vi "IRGetLastLearnedCode.vi"(8 "error in (no error)":errorcluster, 11 "Device In":u64) -> (0 "error out":errorcluster, 1 "codeInfo out":T1={"bitCount"=0, "encoding"=1, "length"=1, "gap"=0, "trail"=0, "header[0]"=0, "header[1]"=0, "one[0]"=0, "one[1]"=0, "zero[0]"=0, "zero[1]"=0, "repeat[0]"=0, "repeat[1]"=0, "repeat[2]"=0, "repeat[3]"=0, "repeat[4]"=0, "repeat[5]"=0, "repeat[6]"=0, "repeat[7]"=0, "repeat[8]"=0, "repeat[9]"=0, "repeat[10]"=0, "repeat[11]"=0, "repeat[12]"=0, "repeat[13]"=0, "repeat[14]"=0, "repeat[15]"=0, "repeat[16]"=0, "repeat[17]"=0, "repeat[18]"=0, "repeat[19]"=0, "repeat[20]"=0, "repeat[21]"=0, "repeat[22]"=0, "repeat[23]"=0, "repeat[24]"=0, "repeat[25]"=0, "minRepeat"=0, "dutyCycle"=0.0, "carrierFrequency"=0, "toggleMask[0]"=0, "toggleMask[1]"=0, "toggleMask[2]"=0, "toggleMask[3]"=0, "toggleMask[4]"=0, "toggleMask[5]"=0, "toggleMask[6]"=0, "toggleMask[7]"=0, "toggleMask[8]"=0, "toggleMask[9]"=0, "toggleMask[10]"=0, "toggleMask[11]"=0, "toggleMask[12]"=0, "toggleMask[13]"=0, "toggleMask[14]"=0, "toggleMask[15]"=0, "toggleMask[16]"=0, "toggleMask[17]"=0, "toggleMask[18]"=0, "toggleMask[19]"=0, "toggleMask[20]"=0, "toggleMask[21]"=0, "toggleMask[22]"=0, "toggleMask[23]"=0, "toggleMask[24]"=0, "toggleMask[25]"=0, "toggleMask[26]"=0, "toggleMask[27]"=0, "toggleMask[28]"=0, "toggleMask[29]"=0, "toggleMask[30]"=0, "toggleMask[31]"=0, "toggleMask[32]"=0} caption="Code Info" {"encoding" items=["IR_ENCODING_UNKNOWN"=1, "IR_ENCODING_SPACE"=2, "IR_ENCODING_PULSE"=3, "IR_ENCODING_BIPHASE"=4, "IR_ENCODING_RC5"=5, "IR_ENCODING_RC6"=6]; "length" items=["IR_LENGTH_UNKNOWN"=1, "IR_LENGTH_CONSTANT"=2, "IR_LENGTH_VARIABLE"=3]}, 2 "Learned Code":string, 3 "Device Out":u64)   [LabVIEW 2012, in "Phidget IR.lvlib"]
doc: "${GetLastLearnedCode:Header}"
uses:
  <instrlib>/Phidgets/Phidget IR/Phidget IR.lvlib
  <instrlib>/Phidgets/Phidget IR/Public/CodeInfo.ctl
  <instrlib>/Phidgets/Phidget Common/Phidget Common.lvlib
  phidget22.dll
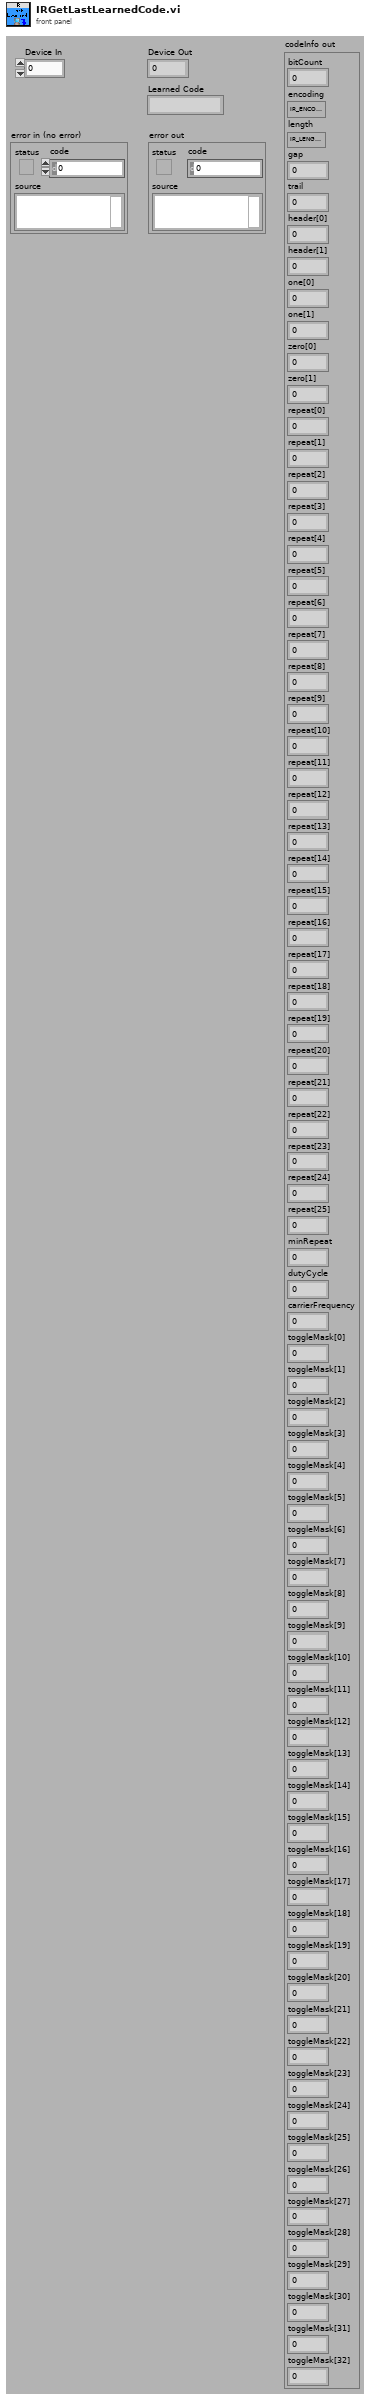
[diagram p1: front panel]
types:
  T1 = typedef "Phidget IR.lvlib/CodeInfo.ctl" = cluster{"bitCount":u32, "encoding":u32, "length":u32, "gap":u32, "trail":u32, "header[0]":u32, "header[1]":u32, "one[0]":u32, "one[1]":u32, "zero[0]":u32, "zero[1]":u32, "repeat[0]":u32, "repeat[1]":u32, "repeat[2]":u32, "repeat[3]":u32, "repeat[4]":u32, "repeat[5]":u32, "repeat[6]":u32, "repeat[7]":u32, "repeat[8]":u32, "repeat[9]":u32, "repeat[10]":u32, "repeat[11]":u32, "repeat[12]":u32, "repeat[13]":u32, "repeat[14]":u32, "repeat[15]":u32, "repeat[16]":u32, "repeat[17]":u32, "repeat[18]":u32, "repeat[19]":u32, "repeat[20]":u32, "repeat[21]":u32, "repeat[22]":u32, "repeat[23]":u32, "repeat[24]":u32, "repeat[25]":u32, "minRepeat":u32, "dutyCycle":dbl, "carrierFrequency":u32, "toggleMask[0]":i8, "toggleMask[1]":i8, "toggleMask[2]":i8, "toggleMask[3]":i8, "toggleMask[4]":i8, "toggleMask[5]":i8, "toggleMask[6]":i8, "toggleMask[7]":i8, "toggleMask[8]":i8, "toggleMask[9]":i8, "toggleMask[10]":i8, "toggleMask[11]":i8, "toggleMask[12]":i8, "toggleMask[13]":i8, "toggleMask[14]":i8, "toggleMask[15]":i8, "toggleMask[16]":i8, "toggleMask[17]":i8, "toggleMask[18]":i8, "toggleMask[19]":i8, "toggleMask[20]":i8, "toggleMask[21]":i8, "toggleMask[22]":i8, "toggleMask[23]":i8, "toggleMask[24]":i8, "toggleMask[25]":i8, "toggleMask[26]":i8, "toggleMask[27]":i8, "toggleMask[28]":i8, "toggleMask[29]":i8, "toggleMask[30]":i8, "toggleMask[31]":i8, "toggleMask[32]":i8}
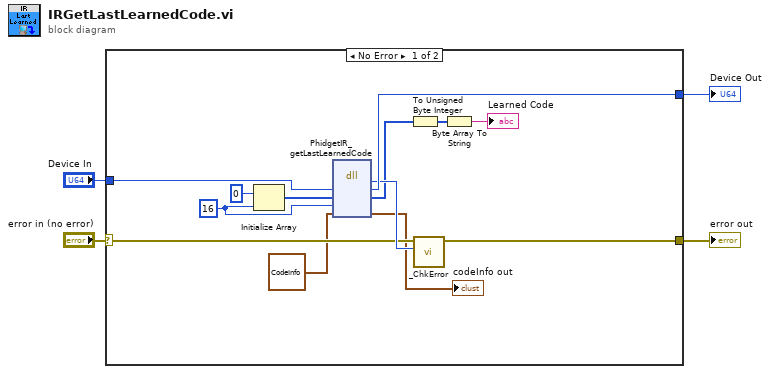
[diagram p0: block diagram]
diagram:
  n1 = case shown="No Error" "error in (no error)" {
    selector: "error in (no error)" -> [w14 w19]
    tunnel: [w13 w19] -> w3
    tunnel: "Device In" -> [w17 w18]
    tunnel: [w16 w18] -> w1
    frame No Error {
      w7 = 16
      n2 = Initialize Array(u8 0, w7) -> (w11:u8[])
      n3 = dll-call lib="phidget22.*" fn="PhidgetIR_getLastLearnedCode"("phid"=w17, "data"=w11, "dataLength"=w7, "codeInfo out"=T1 {"bitCount"=0, "encoding"=1, "length"=1, "gap"=0, "trail"=0, "header[0]"=0, "header[1]"=0, "one[0]"=0, "one[1]"=0, "zero[0]"=0, "zero[1]"=0, "repeat[0]"=0, "repeat[1]"=0, "repeat[2]"=0, "repeat[3]"=0, "repeat[4]"=0, "repeat[5]"=0, "repeat[6]"=0, "repeat[7]"=0, "repeat[8]"=0, "repeat[9]"=0, "repeat[10]"=0, "repeat[11]"=0, "repeat[12]"=0, "repeat[13]"=0, "repeat[14]"=0, "repeat[15]"=0, "repeat[16]"=0, "repeat[17]"=0, "repeat[18]"=0, "repeat[19]"=0, "repeat[20]"=0, "repeat[21]"=0, "repeat[22]"=0, "repeat[23]"=0, "repeat[24]"=0, "repeat[25]"=0, "minRepeat"=0, "dutyCycle"=0.0, "carrierFrequency"=0, "toggleMask[0]"=0, "toggleMask[1]"=0, "toggleMask[2]"=0, "toggleMask[3]"=0, "toggleMask[4]"=0, "toggleMask[5]"=0, "toggleMask[6]"=0, "toggleMask[7]"=0, "toggleMask[8]"=0, "toggleMask[9]"=0, "toggleMask[10]"=0, "toggleMask[11]"=0, "toggleMask[12]"=0, "toggleMask[13]"=0, "toggleMask[14]"=0, "toggleMask[15]"=0, "toggleMask[16]"=0, "toggleMask[17]"=0, "toggleMask[18]"=0, "toggleMask[19]"=0, "toggleMask[20]"=0, "toggleMask[21]"=0, "toggleMask[22]"=0, "toggleMask[23]"=0, "toggleMask[24]"=0, "toggleMask[25]"=0, "toggleMask[26]"=0, "toggleMask[27]"=0, "toggleMask[28]"=0, "toggleMask[29]"=0, "toggleMask[30]"=0, "toggleMask[31]"=0, "toggleMask[32]"=0}) -> ("return type"=w15:i32, "phid"=w16:u64, "data"=w10:u8[], "codeInfo out"=→"codeInfo out":T1)  [unwired: 4 in, 2 out]
      n4 = To Unsigned Byte Integer(number=w10) -> (unsigned 8bit integer=w9:u8[])
      n5 = call <instrlib>:"_ChkError.vi"("Return Code"=w15, "error in (no error)"=w14) -> ("error out"=w13:errorcluster)  [unwired: 9 in]
      n6 = Byte Array To String(unsigned byte array=w9) -> (string=→"Learned Code":string)
    }
    frame Error {
    }
  }
  "error out" <- w3
  "Device Out" <- w1
